vi "ECHOLAB_sweep_BlueMagic_8_LED_robot.vi"() -> ()   [LabVIEW 2014]
uses:
  <vilib>/Analysis/NI_AALBase.lvlib
  <vilib>/Analysis/NI_AALPro.lvlib
  <vilib>/Analysis/2dsp.llb/1D Cross Correlation (DBL).vi
  <vilib>/Analysis/baseanly.llb/Mean (DBL).vi
  <vilib>/DAQmx/write.llb/DAQmx Write (Digital Bool 1Line 1Point).vi
  <vilib>/DAQmx/write.llb/DAQmx Write (Digital 1D Bool NChan 1Samp 1Line).vi
panel:
  out "error out 7":errorcluster
  in  "only one speaker":bool
  in  "Numerisch":i32=6
  in  "Registerkarte":T1(tab)=enum."Statistic"
  in  "?":T2(tab)=enum."Sweep"
  in  "Grundpfad":path=path "C:/Users/Administrator/Documents/New LabView Programms/Aktuelle Programme/Experiment!/Markus/Test_biege_easyIsle"
  in  "Projektname":string="lasttest"
  in  "Lsimp Path":path=path "C:/Users/Administrator/Documents/New LabView Programms/Aktuelle Programme/Experiment!/Markus/Lsimps/Lsimp_EMFI_doubleLayer2"
  out "Projektpfad":path
  in  "EMFI":bool=TRUE
  in  "Sequenz length us":i32=10000
  in  "Sweep Position us":i32=1000
  in  "Fading length us":i32=100
  out "Sweep":waveform(dbl)(graph)={"t0"=timestamp(0 s since 1904-01-01), "dt"=2e-06, "Y"=array[10000 elements]}
  in  "Sweep Dauer us":dbl=3000.0
  in  "Endfrequenz":dbl=30000.0
  in  "Startfrequenz":dbl=160000.0
  in  "Speichern":bool
  out "Active Speaker":bool[](array[boolean])=[FALSE, FALSE, FALSE, FALSE, FALSE, FALSE, FALSE, FALSE, FALSE, FALSE, FALSE, FALSE, TRUE, FALSE]
  out "Current Step":i32=9
  in  "Lautsprecher Winkel 2":dbl[](array[numeric])=[57.5, 62.5, 67.5, 72.5, 77.5, 82.5, 87.5, 92.5, 97.5, 102.5, 107.5, 112.5, 117.5, 122.5]
  in  "?":T3(tab)=enum."Korreliertes Signal 2"
  out "Rohdaten Mic_2":dbl[](graph)
  out "Rohdaten Mic_1":dbl[](graph)
  out "Highpass gefilterte Rohdaten 1":dbl[](graph)
  out "Highpass gefilterte Rohdaten 2":dbl[](graph)
  out "Korreliertes Signal mit richtigem Anfang 1":dbl[](graph)
  out "Mit Sweep korreliert 1":dbl[](graph)
  in  "begin signal 1":dbl=10000.0
  out "Korreliertes Signal mit richtigem Anfang 2":dbl[](graph)
  out "Mit Sweep korreliert 2":dbl[](graph)
  in  "begin signal 2":dbl=10000.0
  out "Verwendete Lsimp":dbl[](graph)=[37.987285423059056, 41.94542933552669, 36.718158358422706, 26.00748307572737, 19.2716180504421, 24.761499073823494, 42.30499601827574, 61.587948563187, 67.89628573083789, 51.70333227535859, 15.399122766613395, -27.68927453387939, -61.37070763335237, -76.15264916698138, -73.86768017091444, -64.72079033459252, -59.52381378965343, -62.88653630335647, -71.76717343532985, -79.45389721021402, -81.22866913949802, -77.36925543013777, -71.79685821069825, -68.16933219563248, -66.83716345038205, -64.88396753245559, -58.77939161586293, -47.22913366886196, -31.960097661366042, -16.007911276056277, -0.957601780562999, 14.83258011472596, 35.88426996664442, 67.42646016772136, 112.61329444376922, 170.32046883201753, 234.13868277323354, 292.7129302295323, 331.46153784141086, 335.73707485805517, 295.22335233505146, 208.6390119317919, 86.97778592958551, -46.80965343474546, -163.0212483502424, -234.6982045240623, -248.3565916317663, -211.17170036320425, -150.16619266006217, -101.95868271871649, -96.40529026626245, -141.58789070049625, -218.28587106890322, -288.03302525625713, -311.67350917905657, -269.0264147906947, -169.00057710982665, -44.606841115389614, 64.01890415431463, 128.6594928873974, 143.66493430186893, 123.6892963416052, 92.1901251937388, 69.13583532468809, 64.83922327141428, 80.91465595446554, 114.10505366272857, 158.17423887163412, 202.9849929659505, 234.17069835907236, 237.13810720723058, 204.90368531355756, 144.26755083610885, 74.11421963653709, 14.839045579973371, -24.61012928577484, -52.16863709716678, -85.0542584663164, -133.37595971808742, -186.99256816490333, -216.89265836020712, -192.62474702620085, -105.2705475364944, 19.88830084818578, 131.07229196653836, 174.9072799253783, 123.9788348833058, -9.122072661395347, -178.45784850808047, -326.4793694986597, -407.4491440952962, -400.941475403144, -312.31821988357115, -165.1330278590582, 7.545121930961784, 169.73077975035375, 288.6320105760493, 342.59757383091426, 329.43731496614197, 269.5355622823815, 198.62746495525653, 151.1277946685444, 142.28248330950265, 160.03536063923315, 172.48295121369566, 147.08158850809662, 70.14025726278376, -44.961580421148035, -164.9711932091802, -253.9338579639399, -289.68706855950416, -271.08402995295086, -214.24499349508537, -142.51142765887988, -76.62533165610529, -29.048182137794647, -2.5152144966053003, 8.879387744009524, 16.999498652431683, 35.028807650487735, 70.9591859098809, 121.51231551074474, 170.52550094534286, 194.6168672600115, 174.70853553953242, 107.51186045471589, 9.93561022984685, -87.01517468482572, -152.02697733843473, -167.43181691881233, -135.84534566440934, -76.63424130617673, -15.304023561933974, 27.73181681265263, 43.48100822634696, 34.20774270023911, 9.028054419071426, -21.094648548475305, -46.562847934060166, -60.39229615626998, -58.61648097387942, -40.720888785491965, -9.95678133454292, 27.198727840329127, 62.78429492138909, 89.75636837754168, 103.97627526024421, 104.94515156439942, 95.17354586658846, 78.67523010824826, 59.256086140600914, 39.14916197776178, 18.419707567058776, -4.53429131695286, -31.359167324869112, -61.60716713863444, -91.31357632662373, -113.5222858413143, -121.02690136101434, -110.10016494050913, -83.00220288733615, -47.49118008118892, -13.322545050646244, 12.316883061252692, 27.737392500670154, 36.38229758518521, 43.65244700708752, 53.12187538151082, 64.48349513224547, 74.14700753033969, 77.60736295621001, 71.80331292821236, 56.17513240504583, 32.37375911823534, 3.4627367567873555, -26.62897321273065, -53.397178059119526, -72.34957116923633, -80.22839594278574, -76.41884765260448, -63.53246629100458, -46.440467539101725, -30.051069869735283, -17.082827718919397, -7.188938774909889, 2.0994401876032778, 13.343105063752096, 27.432584546910252, 43.08171772566773, 57.587134526822325, 68.0662292444963, 72.33213728362517, 69.13204626316582, 58.08493838266445, 39.7682572566104, 16.002080433379952, -10.069811728438523, -34.5306095944581, -53.8364889717854, -65.97272873380305, -70.90309347902996, -70.02677876043627, -65.03196685626713, -56.90758277963846, -45.69501643915526, -31.00235289689016, -12.805913828058124, 8.013068875792442, 29.644160069832875, 49.706586339083785, 65.72366452061605, 75.56557454467972, 77.8751474823423, 72.48313804653267, 60.64901799215318, 44.85647944539737, 28.053216272045916, 12.592101934969236, -0.5703833046869773, -11.92788800291775, -22.68227095779246, -33.678613480551, -44.69092768297345, -54.460430330636825, -61.351280097982695, -64.10659971309258, -62.226391914044754, -55.86269279903715, -45.52248460302857, -31.930615670932838, -16.144321341606098, 0.3192571896456796, 15.651291021180189, 28.259121968674897, 37.307148605525796, 42.86896311084485, 45.52674876328166, 45.68907117249621, 43.1533923702947, 37.285299525259305, 27.717818644463748, 15.063835342580322, 1.09861362859763, -11.761034684139855, -21.362230547589427, -26.545860965660452, -27.311966112040114, -24.449178789685256, -18.98880063520781, -11.859596605121695, -3.8566927215703863, 4.246542650360977, 11.681910293034626, 17.83766248205442, 22.428960778401663, 25.480209919729468, 27.078861865530516, 27.08775142595211, 25.082005453718555, 20.611753000725564, 13.626659246561587, 4.7425311670550885, -4.869942969188056, -13.919586156575697, -21.471781523790362, -27.177548910451407, -31.16182125158828, -33.71583021036854, -35.03910551569061, -35.16954647736422, -34.06207997379421, -31.669590588025734, -27.936554105228137, -22.75141917097973, -15.980520596397886, -7.639329094944579, 1.8899819246897778, 11.769595911840018, 20.859044110038674, 28.056029628887828, 32.627847523818204, 34.35154124141151, 33.42281412422663, 30.256602385756544, 25.346837423716195, 19.256450690601064, 12.661021482984339, 6.318294154753728, 0.912547672939884, -3.13874461051835, -5.76817117503621, -7.15697915173641, -7.522403709934467, -6.960713149988033, -5.465938798812448, -3.0917352098321413, -0.09624096730401532, 3.0748575670448757, 5.970285329410185, 8.33003766291407, 10.126408347639087, 11.40559072656139, 12.06406962932657, 11.756856138530953, 10.033353177332586, 6.611505107116842, 1.5840530992770214, -4.594870237638631, -11.322520610248993, -18.082087377026, -24.521473842257514, -30.34447353803086, -35.150092644557205, -38.400157160262964, -39.57989702216926, -38.43148546041212, -35.06667472234177, -29.850930108971063, -23.142794630831233, -15.106002216192778, -5.765961157179861, 4.719486173324453, 15.78972267144523, 26.45011877168526, 35.54746915313663, 42.18800189416256, 46.024055317696046, 47.23280922339901, 46.23648737352134, 43.39003268668904, 38.85941230891154, 32.74295226898982, 25.29262513752641, 17.025656379837578, 8.623949422155569, 0.7042607056616654, -6.355400409638805, -12.406264834922581, -17.370160143207055, -21.092711794336847, -23.35391752325315, -24.03506410806453, -23.295367971810453, -21.592699300181494, -19.50292468346278, -17.45795729745628, -15.591256485359558, -13.80111204093922, -11.971363960105585, -10.17454538585567]
  out "error out 2":errorcluster
  in  "Datenbank? R1-M1":bool=TRUE
  in  "Datenbank? R1-M2":bool=TRUE
  in  "Datenbank? R2-M1":bool=TRUE
  in  "Datenbank? R2-M2":bool=TRUE
  in  "Datenbank? R3-M1":bool=TRUE
  in  "Datenbank? R3-M2":bool=TRUE
  in  "Pfad? R1-M1":path=path "C:/Users/Administrator/Documents/New LabView Programms/Aktuelle Programme/Experiment!/HuanSubVIs/S70-21_M1.csv"
  in  "Pfad? R1-M2":path=path "C:/Users/Administrator/Documents/New LabView Programms/Aktuelle Programme/Experiment!/HuanSubVIs/S70-21_M2.csv"
  in  "Pfad? R2-M1":path=path "C:/Users/Administrator/Documents/New LabView Programms/Aktuelle Programme/Experiment!/HuanSubVIs/S50-20_M1.csv"
  in  "Pfad? R2-M2":path=path "C:/Users/Administrator/Documents/New LabView Programms/Aktuelle Programme/Experiment!/HuanSubVIs/S50-20_M2.csv"
  in  "Pfad? R3-M1":path=path "C:/Users/Administrator/Documents/New LabView Programms/Aktuelle Programme/Experiment!/HuanSubVIs/S35-10_M1.csv"
  in  "Pfad? R3-M2":path=path "C:/Users/Administrator/Documents/New LabView Programms/Aktuelle Programme/Experiment!/HuanSubVIs/S35-10_M2.csv"
  in  "Gap Refl2 (samples)":dbl=62.0
  in  "Gap Refl1 (samples)":dbl=85.0
  in  "Gap Refl3 (samples)":dbl=41.0
  in  "MaxtPeak miltiplication \nfactor -R1":dbl=15.0
  in  "MaxtPeak miltiplication\n factor R3":dbl=25.0
  in  "MaxtPeak miltiplication\n factor -R2":dbl=50.0
  in  "Grenz Ampulitude-R3":dbl=80.0
  in  "Grenz Ampulitude-R1":dbl=100.0
  in  "Grenz Ampulitude-R2":dbl=100.0
  out "Refl_1":dbl[][](graph)
  out "Refl_3":dbl[][](graph)
  in  "Stopabstand 1":dbl=30.0
  out "Max. Wert Refl_1":dbl=0.00024072035967195873
  in  "Stopabstand 2":dbl=30.0
  out "Abstand-Array-Refl 2":dbl=38.09710163220162
  in  "turn left/right?":bool=TRUE
  out "Max. Wert Refl_2":dbl=0.0023395203738088097
  in  "Stopabstand 3":dbl=30.0
  out "Abstand-Array-Refl 3":dbl=62.91468799787438
  in  "LED turn on?":bool=TRUE
  out "Max. Wert Refl_3":dbl=0.0018103910057642178
  out "probability":dbl[][](graph)=[[3.0000000000000004e-05, 5.000000000000001e-05, 7.000000000000001e-05, 9e-05, 0.00011, 0.0001300124738367786, 0.00023072035967195873, 0.00025072035967195873], [3.0000000000000004e-05, 5.000000000000001e-05, 7.000000000000001e-05, 9e-05, 0.0017493906595402342, 0.0017803910057642178, 0.0018003910057642178, 0.0018203910057642179], [0.00038194151602209035, 0.0009686688450150448, 0.0022439203760585267, 0.004143838935916074, 0.005245931301535438, 0.005272342187251083, 0.002320526795117191, 0.0023585139525004284]]
  out "probability/distance":dbl[][](graph)=[[1.8750000000000003e-06, 5.891036022775227e-06, 6.000006000006e-11, 8.000008000008e-11, 1.0000010000010001e-10, 3.239128915113618e-06, 4.868667316483549e-06, 8.424336383279796e-06], [1.8750000000000003e-06, 5.891036022775227e-06, 6.000006000006e-11, 8.000008000008e-11, 1.185535180537081e-05, 2.5560005321415227e-05, 2.593027246994507e-05, 2.9887064473399943e-05], [5.616787000324858e-06, 1.1108824384371127e-05, 3.0643367217874765e-05, 7.270750187692021e-05, 0.0001283583707298027, 0.00018749870693041687, 9.480098082220174e-05, 6.766626049238367e-05]]
  in  "robotControl":bool
  out "Actions?":bool=TRUE
  in  "x links Refl1":i32=200
  in  "y links Refl1":i32=500
  out "x/y":dbl=1e-05
  out "gefahrene (cm)":dbl=59.86920617947912
  out "time diff (s)":dbl=3.314115524291992
  out "gefahren(mm)":dbl=84.43606431317178
  in  "Velocity":dbl=4000.0 format="%#_13g"
  in  "origin Y(cm)":dbl=-10.0 format="%#_13g"
  in  "Velocity (mm per sec)":dbl=40.0 format="%#_13g"
  in  "robot aktiv":bool
  in  "Lineareinheit aktiv":bool=TRUE
  in  "x-move (mm)":dbl=8000.0
  out "R1-Action":bool
  out "R2-Action":bool
  out "R3-Action":bool
  out "Abstand-Array-Refl1":dbl=28.64430745806648
  in  "Sigma-R3":dbl=1.8
  in  "Sigma-R2":dbl=1.5
  in  "Sigma-R1":dbl=1.0
  out "Abstand-Array-Refl3\n(in y Richtung)":dbl=60.57440025183806
  out "Abstand-Array-Refl2\n(in y Richtung)":dbl=34.57440025183806
  out "Abstand-Array-Refl1\n(in y Richtung)":dbl=28.574400251838057
  out "y_R3":i32=112
  out "x_R3":i32=83
  out "y_R1":i32=80
  out "x_R1":i32=102
  out "y_R2":i32=86
  out "x_R2":i32=82
  out "Refl_2":dbl[][](graph)
  out "Signalverlaufsgraph 3":dbl[][](graph)
  out "korriliertes Singnal":dbl[](graph)
  in  "Mic. 1      /      Mic. 2":bool
  in  "LS auswählen":i32=11
  in  "Standard Gap eingeben":dbl=85.0
  out "Locations":dbl[](array[numeric])
  out "distanceMatrix":dbl[][](array[numeric])
  out "Array 2":dbl[](array[numeric])
  out "HS":bool
  in  "MaxtPeak miltiplication factor":dbl=50.0
  in  "Stopp 2":bool
  in  "Message":string="60;0;15"
  out "error out 6":errorcluster
  out "error out 5":errorcluster
  # "Nein"
  # "Ja"
  # "1     2     3     4     5     6     7     8     9    10   11   12   13   14"
  # "Polaroid"
  # "orange 70 mm"
  # "blau 50 mm"
  # "gruen 35 mm"
  # "green"
  # "orange"
  # "blau"
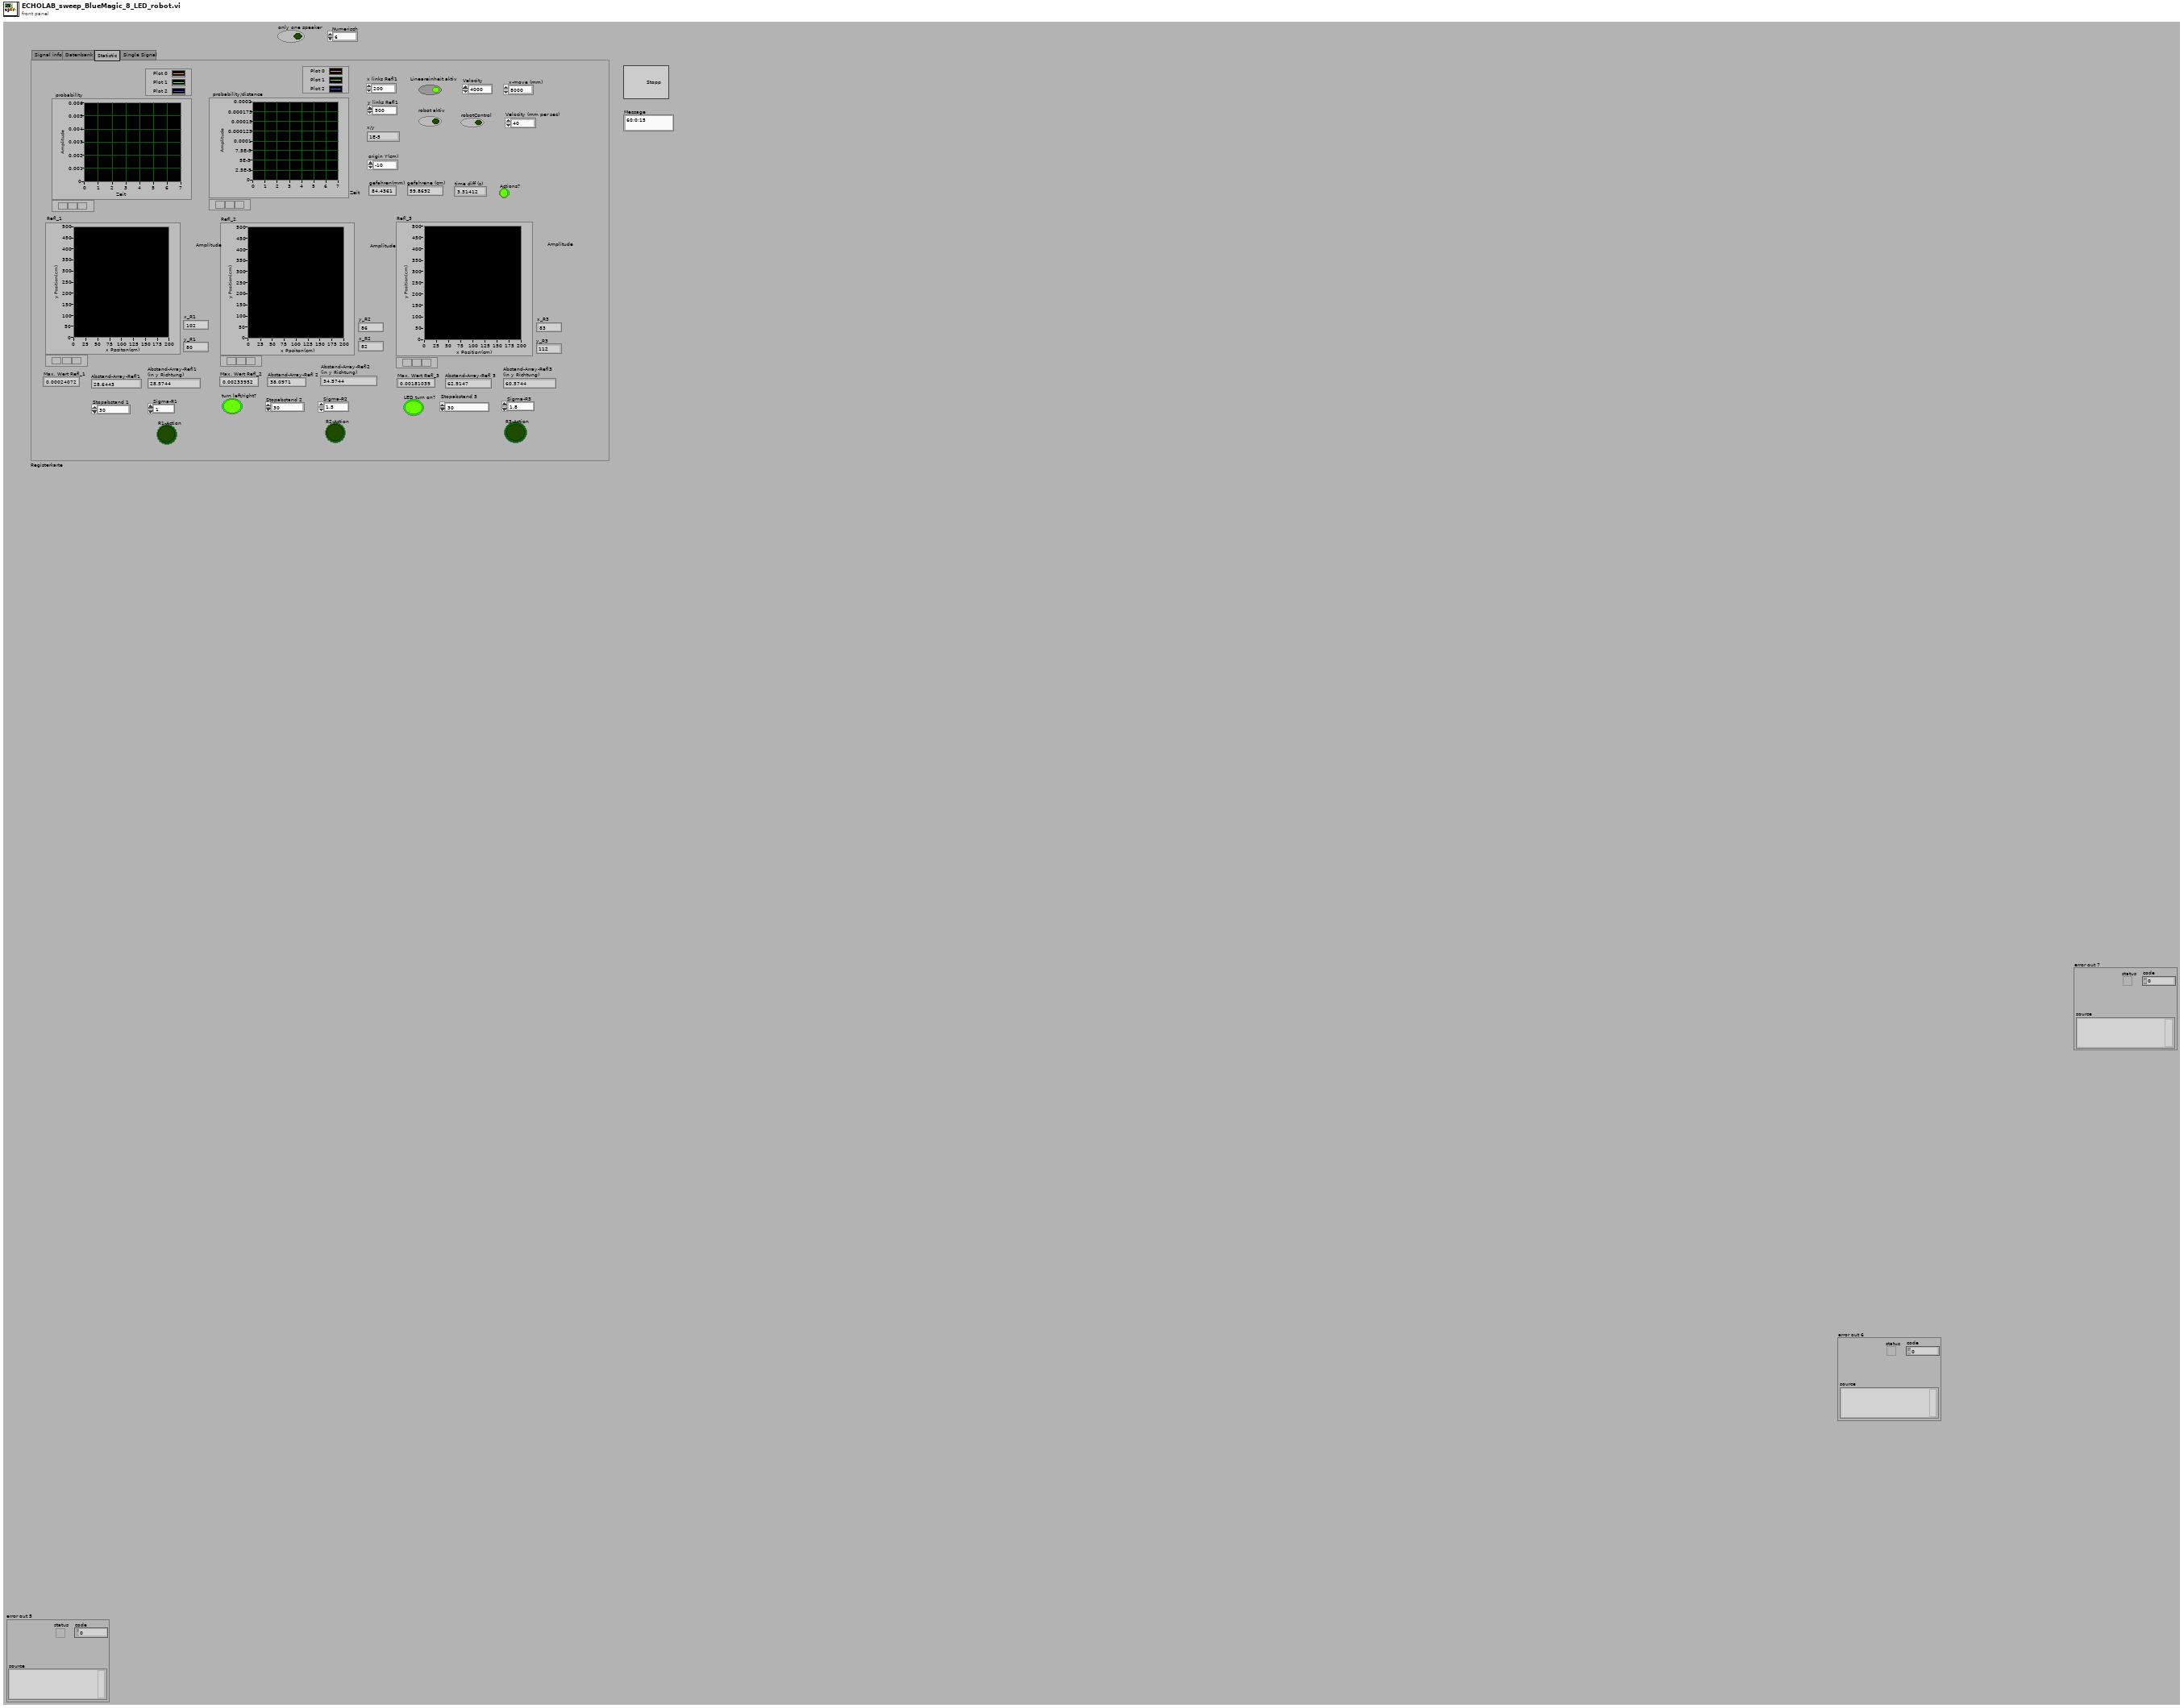
[diagram p1: front panel]
types:
  T1 = enum32{"Signal info", "Datenbank", "Statistic", "Single Signal"}
  T2 = enum32{"Daten einlesen und speichern", "Sweep", "HK", "Winkel & Korrektur"}
  T3 = enum32{"Rohdaten", "Rohdaten HP", "Korreliertes Signal 1", "Korreliertes Signal 2", "Intensity Graphs", "Lsimp", "Errors"}
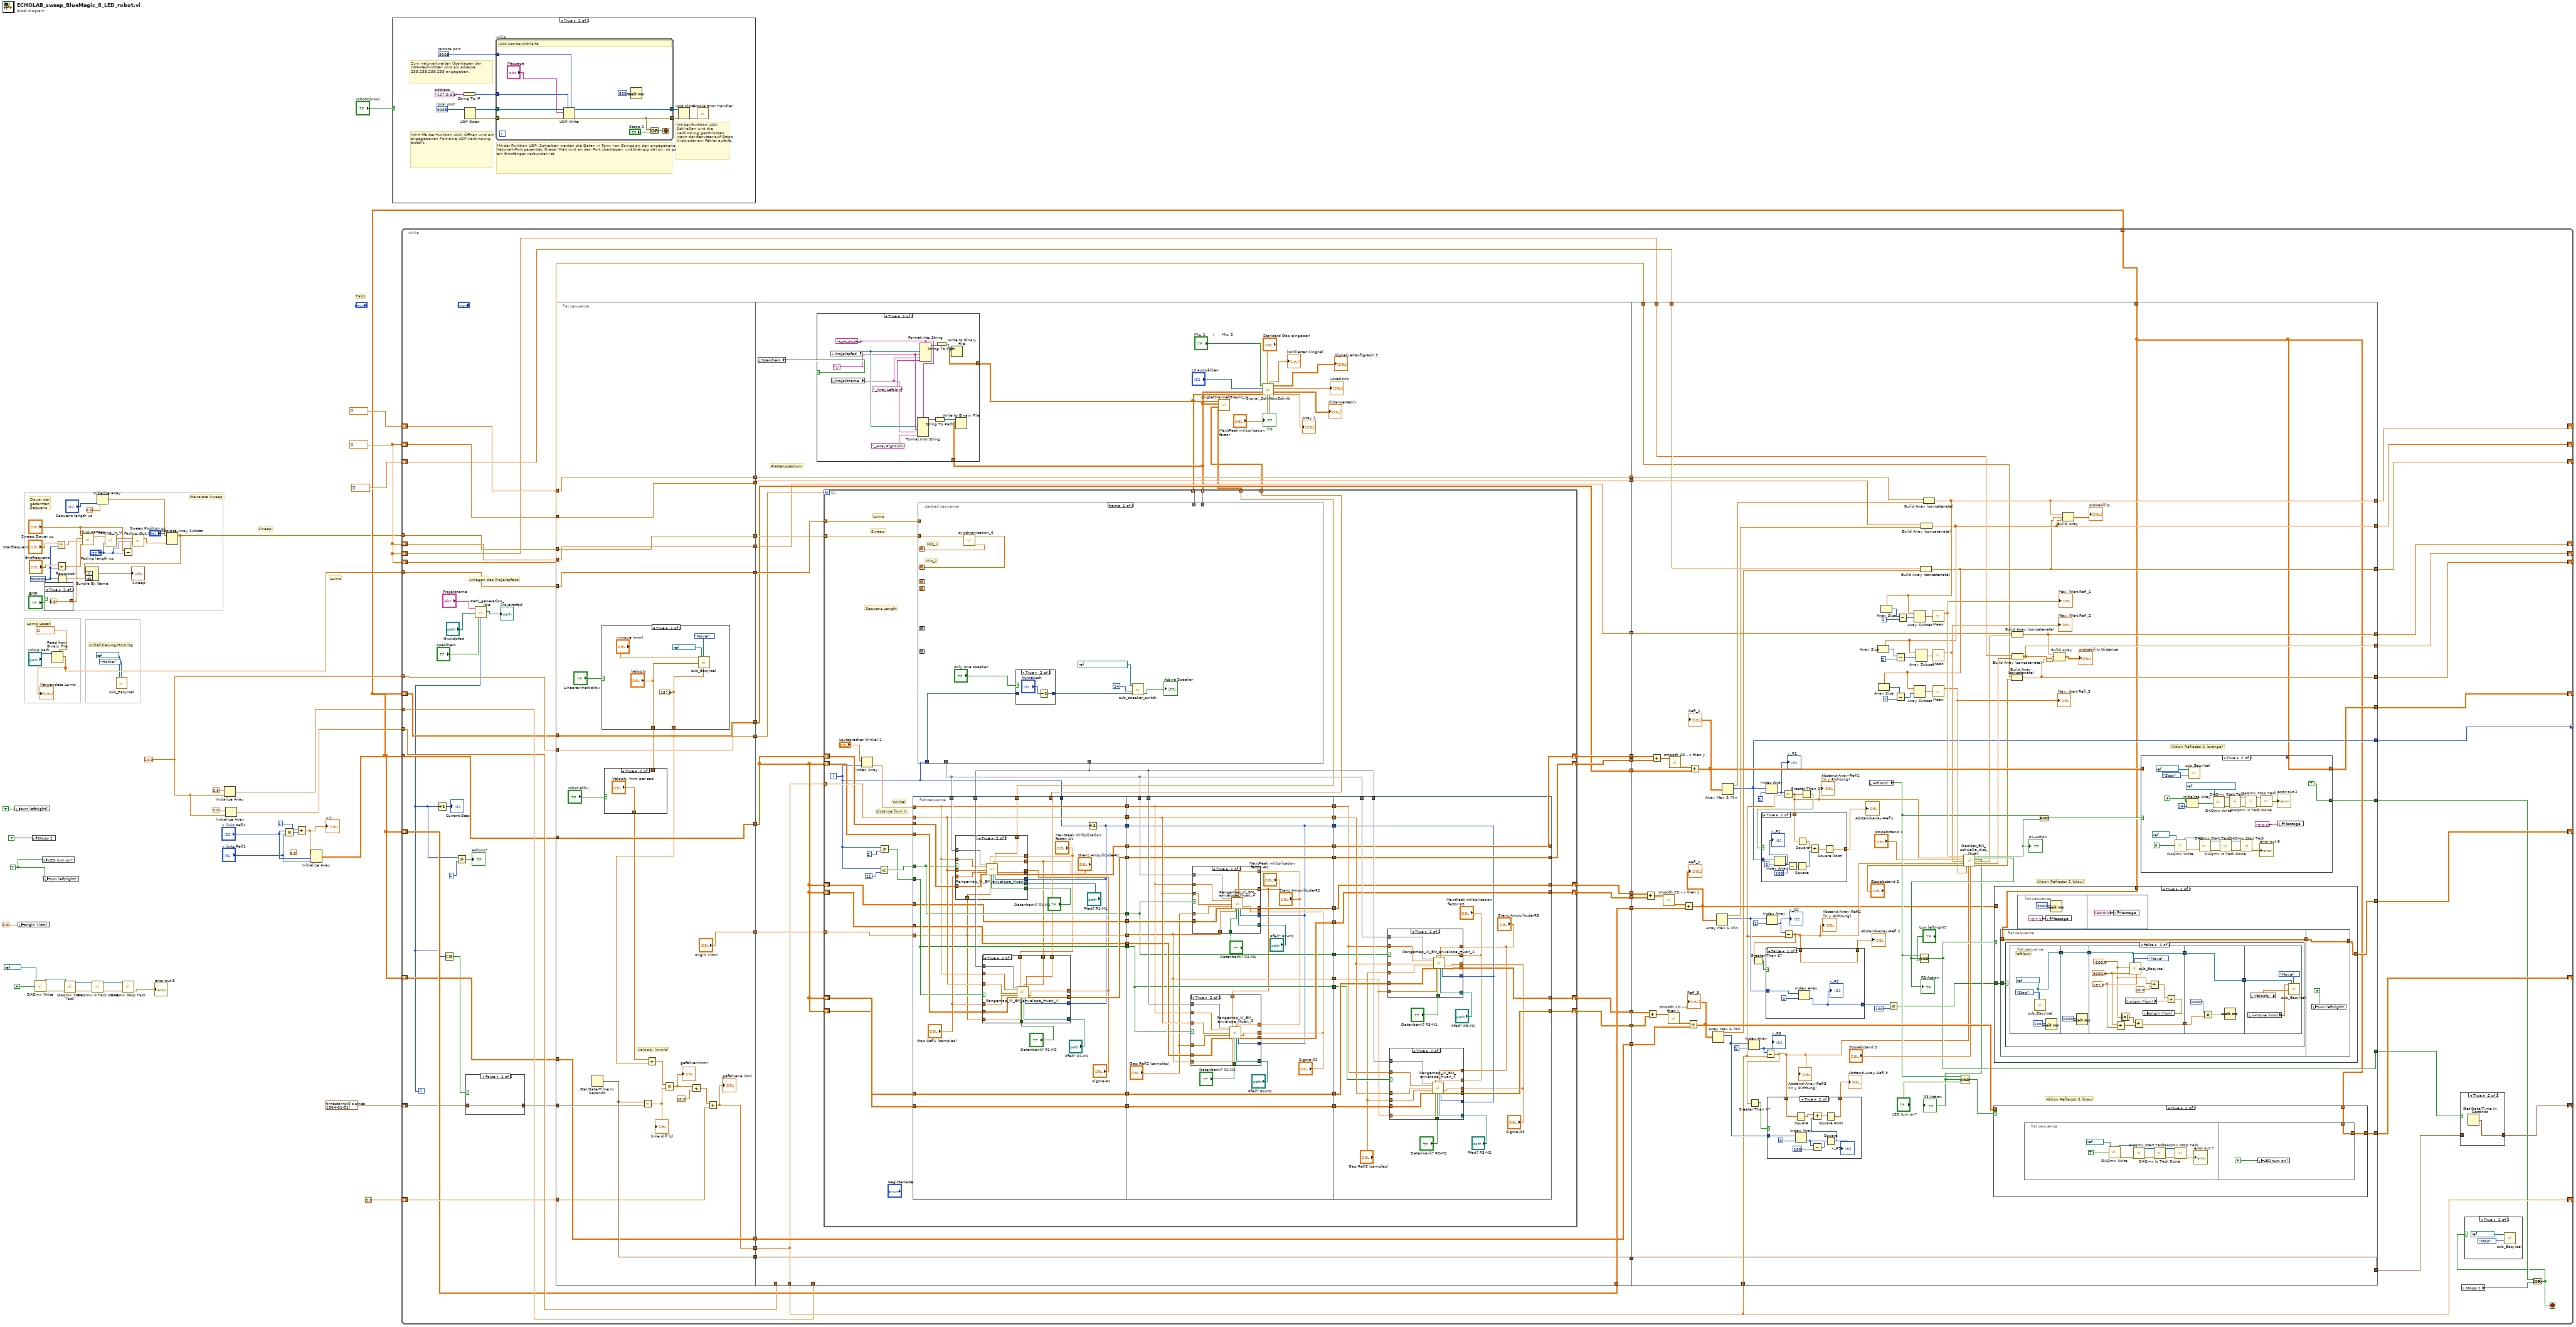
[diagram p0: block diagram]
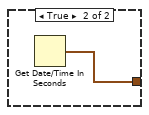
[diagram p5: hidden frame]
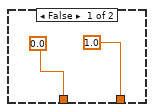
[diagram p7: hidden frame]
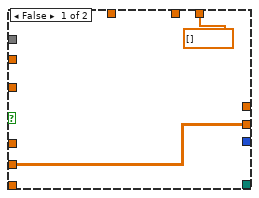
[diagram p9: hidden frame]
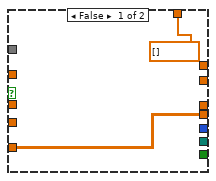
[diagram p10: hidden frame]
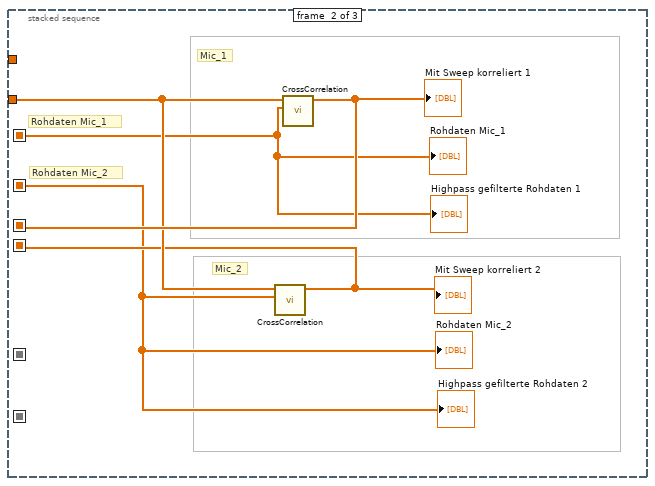
[diagram p16: hidden frame]
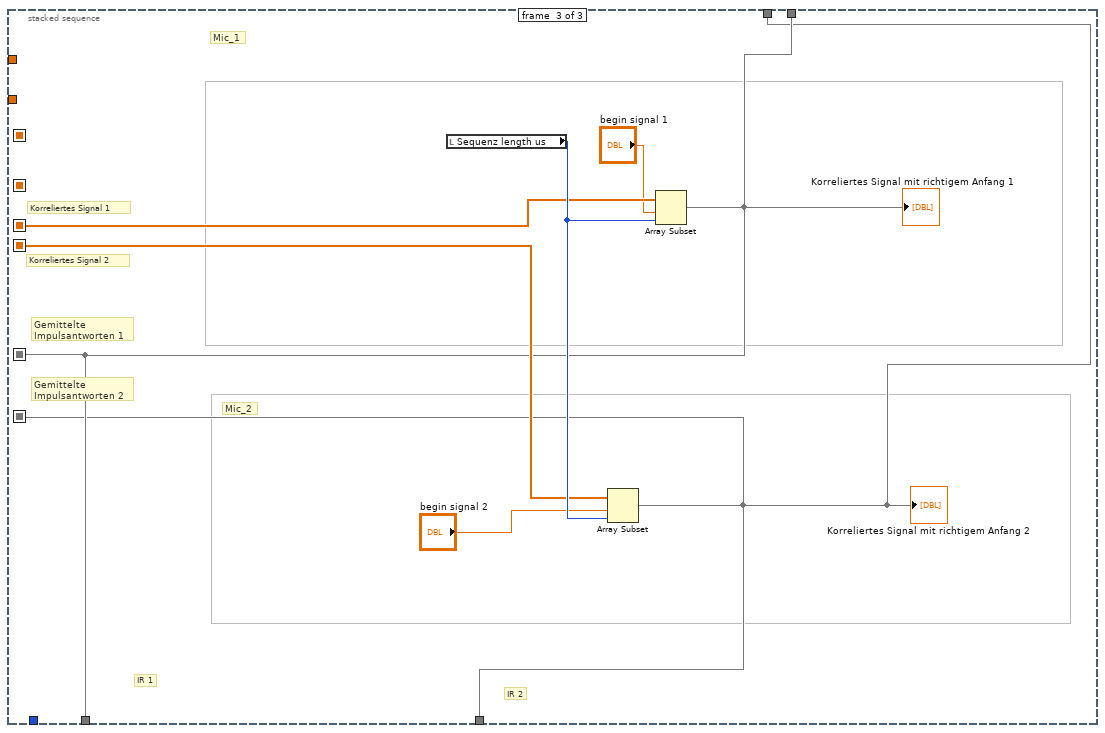
[diagram p17: hidden frame]
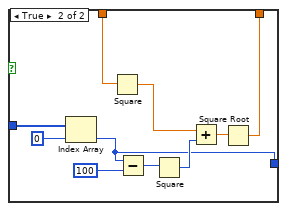
[diagram p19: hidden frame]
diagram:
  w15 = dbl[] []
  w21 = TRUE
  (unwired) 0.0 ("Element")
  w30 = 14.0 ("Anzahl Lautsprecher")
  w48 = 500000
  # "Sweep"
  # "Lsimp"
  # "Initialisierung/Homing"
  # "Dauer der\ngesamten\nSequenz"
  # "Generate Sweep"
  # "Tabs"
  # "Lsimp Lesen"
  n1 = local write "turn left/right?"(TRUE ("x < y?")) -> ()
  n2 = local write "origin Y(cm)"(0.0 ("origin(cm) Y")) -> ()
  n3 = local write "Stopp 2"(FALSE) -> ()
  n4 = call-poly <vilib>:"DAQmx Write.vi"("task/channels in"=refnum<k21> "LED", "data"=FALSE) -> ("task out"=w14:refnum<k21>, "error out"=w13:errorcluster)  [unwired: 11 in, 1 out]
  n5 = local write "LED turn on?"(w21) -> ()
  n6 = local write "turn left/right?"(w21) -> ()
  n7 = case shown="True" "EMFI" {
    tunnel: [1 9.0 ("amplitude")] -> w34
    frame False {
    }
    frame True {
    }
  }
  n8 = Read from Binary File(5:dbl[] [], 11:"Lsimp Path") -> (2:w53:dbl[])  [unwired: 4 in, 3 out]
  "Verwendete Lsimp" <- w53
  n9 = Divide(x="Startfrequenz", y=w48) -> (x/y=w51:dbl)
  n10 = Divide(x="Endfrequenz", y=w48) -> (x/y=w49:dbl)
  n11 = Reciprocal(x=w48) -> (1/x=w47:dbl)
  n12 = call <vilib>:"DAQmx Start Task.vi"("task/channels in"=w14, "error in"=w13) -> ("task out"=w12:refnum<k21>, "error out"=w11:errorcluster)  [unwired: 12 in]
  n13 = call <vilib>:"Chirp Pattern.vi"("f2"=w49, "f1"=w51, "amplitude"=w34, "samples"="Sweep Dauer us") -> ("Chirp Pattern"=w44:dbl[])  [unwired: 1 out]
  n14 = call <vilib>:"DAQmx Is Task Done.vi"("task/channels in"=w12, "error in"=w11) -> ("task out"=w10:refnum<k21>, "error out"=w9:errorcluster)  [unwired: 11 in, 1 out]
  n15 = Initialize Array(0.0 ("element"), "Sequenz length us") -> (w43:dbl[])
  n16 = call "Fading_In_VI.vi"("Input Array"=w44, "Fading Index"="Fading length us") -> ("Rising Array"=w42:dbl[])  [unwired: 12 in, 1 out]
  n17 = call "sub_EasyIsel.vi"("VISA resource name"=refnum<visa-resource-name> "COM4", "Mode"=enum16{"Position", "Move", "Stop", "Home"}."Home") -> ()  [unwired: 14 in, 4 out]
  n18 = Subtract(x="Sweep Dauer us", y="Fading length us") -> (x-y=w40:dbl)
  n19 = call <vilib>:"DAQmx Stop Task.vi"("task/channels in"=w10, "error in"=w9) -> ("error out"=→"error out 5":errorcluster)  [unwired: 12 in, 1 out]
  n20 = call "Fading_Out_VI.vi"("Input Array"=w42, "Fading length"="Fading length us", "Fading Index"=w40) -> ("Faded Array"=w41:dbl[])  [unwired: 11 in, 1 out]
  n21 = Replace Array Subset(array=w43, new element=w41, index="Sweep Position us") -> (w4:dbl[])
  n22 = Bundle By Name("Y"=w4, "dt"=w47) -> (→"Sweep":waveform(dbl))  [unwired: 1 in]
  n23 = Initialize Array(0.0, w30) -> (w32:dbl[])
  n24 = Initialize Array(0.0, w30) -> (w29:dbl[])
  n25 = Multiply(x="x links Refl1", y="y links Refl1") -> (x*y=w27:i32)
  n26 = Divide(x=1, y=w27) -> (x/y=w23:dbl)
  "x/y" <- w23
  n27 = Initialize Array(w23, "x links Refl1", "y links Refl1") -> (w17:dbl[][])
  n28 = case shown="True" "robotControl" {
    frame False {
    }
    frame True {
      w58 = u16 5005  # remote port
      w59 = u16 5005  # local port
      w64 = "127.0.0.1"  # address
      # "Zum netzwerkweiten Übertragen der UDP-Nachrichten wird als Adresse 255.255.255.255 angegeben."
      # "Mit der Funktion UDP: Schließen wird die Verbindung geschlossen, wenn der Benutzer auf Stopp klickt oder ein Fehler auftritt."
      # "Mit der Funktion UDP: Schreiben werden die Daten in Form von Strings an den angegebenen Netzwerk-Port gesendet. Dieser Wert wird an den Port übertragen, unabhängig davon, ob gerade ein Empfänger verbunden ist."
      # "Mit Hilfe der Funktion UDP: Öffnen wird am angegebenen Port eine UDP-Verbindung erstellt."
      n29 = String To IP(1:w64) -> (0:w62:u32)
      n30 = UDP Open(11:w59) -> (port=w61:refnum<k16>, 0:w60:errorcluster)  [unwired: 4 in, 1 out]
      n31 = while {
        tunnel: [w71] -> w65
        tunnel: w61 -> [w76]
        tunnel: w60 -> [w75]
        tunnel: [w72] -> w66
        tunnel: w62 -> [w70]
        tunnel: w58 -> [w68]
        stop <- w74 stop-if-true
        # "UDP-Sender-Schleife"
        n32 = UDP Write(address=w70, port or service name=w68, connection ID=w76, data in="Message", 8:w75) -> (error out=w71:errorcluster, 3:w72:refnum<k16>)  [unwired: 1 in]
        n33 = Wait (ms)(milliseconds to wait=u32 500) -> ()  [unwired: 1 out]
        n34 = Or(x=w71, y="Stopp 2") -> (x .or. y?=w74:bool)
      }
      n35 = UDP Close(connection ID=w66, 8:w65) -> (error out=w63:errorcluster)  [unwired: 1 out]
      n36 = call <vilib>:"Simple Error Handler.vi"("error in (no error)"=w63) -> ()  [unwired: 4 in, 5 out]
    }
  }
  n37 = while {
    tunnel: w30 -> [w141]
    tunnel: w53 -> [w146]
    tunnel: w4 -> [w87]
    tunnel: w32 -> [w142]
    tunnel: w29 -> [w140]
    shift-right: [w97] -> _
    shift-left: timestamp(0 s since 1904-01-01) ("seconds since 1Jan1904") -> [w102]
    shift-right: [w81] -> _
    shift-left: 0.0 -> [w134]
    tunnel: [w83] -> _ mode=indexing
    shift-right: [w86] -> _
    shift-left: w17 -> [w117]
    shift-right: [w126] -> _
    shift-left: dbl[] [] -> [w127]
    shift-right: [w128] -> _
    shift-left: w15 -> [w125]
    tunnel: w17 -> [w119]
    shift-right: [w116] -> _
    shift-left: w17 -> [w114]
    shift-right: [w85] -> _
    shift-left: w17 -> [w110]
    shift-right: [w105] -> _
    shift-left: dbl[] [] -> [w104]
    tunnel: w17 -> [w100]
    shift-right: [w82] -> _
    shift-left: w15 -> [w94]
    shift-right: [w96] -> _
    shift-left: w15 -> [w91]
    shift-right: [w95] -> _
    shift-left: w15 -> [w90]
    i -> [w88]
    stop <- w78 stop-if-true
    # "Anlegen des Projektpfads"
    n38 = Increment(x=w88) -> (x+1=→"Current Step":i32)
    n39 = Equal To 0?(x=w88) -> (x = 0?=w103:bool)
    n40 = Greater?(x=w88, y=1) -> (0:→"Actions?":bool)
    n41 = case shown="False" w103 {
      tunnel: w102 -> [w151 _]
      tunnel: [w151 w152] -> w101
      frame False {
      }
      frame True {
        n42 = Get Date/Time In Seconds() -> (seconds since 1Jan1904=w152:timestamp)
      }
    }
    n43 = call "Path_generation_isle.vi"("Projektname"="Projektname", "Basis-Pfad"="Grundpfad", "Pfad erstellen ? [T]"="Speichern", "Revison"=w88) -> ("Erstellter Pfad"=→"Projektpfad":path)  [unwired: 11 in, 4 out]
    n44 = flat-sequence {
      tunnel: w87 -> [w174]
      tunnel: w146 -> [w175]
      tunnel: w141 -> [w176]
      tunnel: [w176] -> w145
      tunnel: [w175] -> w144
      tunnel: [w174] -> w143
      tunnel: [w170] -> w137
      tunnel: w101 -> [w169]
      tunnel: [w153] -> w135
      tunnel: w134 -> [w155]
      tunnel: w127 -> [w167]
      tunnel: w125 -> [w166]
      tunnel: [w167] -> w124
      tunnel: [w166] -> w122
      tunnel: [w165] -> w120
      tunnel: w119 -> [w165]
      tunnel: [w164] -> w115
      tunnel: w114 -> [w164]
      tunnel: w110 -> [w163]
      tunnel: [w163] -> w109
      tunnel: ["origin Y(cm)"] -> w99
      tunnel: w94 -> [w161]
      tunnel: [w161] -> w93
      tunnel: w145 -> [w215]
      tunnel: w144 -> [w219]
      tunnel: w143 -> [w214]
      tunnel: w142 -> [_]
      tunnel: w140 -> [_]
      tunnel: [w217] -> w139
      tunnel: [w216] -> w138
      tunnel: w137 -> [w190]
      tunnel: [w190] -> w136
      tunnel: w135 -> [w191]
      tunnel: [w213] -> w130
      tunnel: [w200] -> w129
      tunnel: w124 -> [w212]
      tunnel: [w212] -> w123
      tunnel: w122 -> [w211]
      tunnel: [w211] -> w121
      tunnel: w120 -> [w205]
      tunnel: [w210] -> w118
      tunnel: w117 -> [w210]
      tunnel: w115 -> [w209]
      tunnel: [w209] -> w113
      tunnel: [w208] -> w112
      tunnel: [w207] -> w111
      tunnel: w109 -> [w206]
      tunnel: [w206] -> w108
      tunnel: w99 -> [w204]
      tunnel: w93 -> [w203]
      tunnel: [w203] -> w92
      tunnel: [w191] -> w81
      tunnel: w139 -> [w503]
      tunnel: w138 -> [w557]
      tunnel: w136 -> [w523]
      tunnel: [w523] -> w98
      tunnel: w81 -> [w486]
      tunnel: w130 -> [w560]
      tunnel: w129 -> [w502]
      tunnel: [w529] -> w126
      tunnel: [w474] -> w128
      tunnel: w123 -> [w562]
      tunnel: w121 -> [w561]
      tunnel: [w526] -> w86
      tunnel: w118 -> [w501]
      tunnel: [w527] -> w116
      tunnel: w113 -> [w554]
      tunnel: w112 -> [w550]
      tunnel: w111 -> [w549]
      tunnel: [w524] -> w85
      tunnel: w108 -> [w546]
      tunnel: [w473] -> w105
      tunnel: w104 -> [w545]
      tunnel: w100 -> [w472]
      tunnel: [w508] -> w82
      tunnel: [w476] -> w96
      tunnel: [w475] -> w95
      tunnel: w92 -> [w507]
      tunnel: w91 -> [w477]
      tunnel: w90 -> [w506]
      tunnel: [w505] -> w84
      tunnel: [w485] -> w83
      tunnel: [w498] -> w79
      frame #0 {
        # "Velocity (mm/s)"
        n45 = Get Date/Time In Seconds() -> (seconds since 1Jan1904=w170:timestamp)
        n46 = case shown="True" "Lineareinheit aktiv" {
          tunnel: [0.0 "Velocity"] -> w158
          tunnel: [1.0 w182] -> w156
          frame False {
          }
          frame True {
            w182 = 157.0 ("Steps/mm (x)")
            n47 = call "sub_EasyIsel.vi"("x-Position"="x-move (mm)", "Velocity (x)"="Velocity", "VISA resource name"=refnum<visa-resource-name> "COM4", "Mode"=enum16{"Position", "Move", "Stop", "Home"}."Move", "Steps/mm (y)"=w182) -> ()  [unwired: 11 in, 4 out]
          }
        }
        n48 = case shown="True" "robot aktiv" {
          tunnel: w158 -> [w177 _]
          tunnel: [w177 "Velocity (mm per sec)"] -> w157
          frame False {
          }
          frame True {
          }
        }
        n49 = Subtract(x=w170, y=w169) -> (x-y=w173:dbl)
        "time diff (s)" <- w173
        n50 = Divide(x=w157, y=w156) -> (x/y=w154:dbl)
        n51 = Multiply(x=w154, y=w173) -> (x*y=w172:dbl)
        "gefahren(mm)" <- w172
        n52 = Divide(x=w172, y=10.0) -> (x/y=w168:dbl)
        n53 = Add(x=w168, y=w155) -> (x+y=w153:dbl)
        "gefahrene (cm)" <- w153
      }
      frame #1 {
        # "Plattenspektrum"
        n54 = local read "Speichern"() -> (w218:bool)
        n55 = for {
          N: w215 -> [_]
          tunnel: w219 -> [w284]
          tunnel: w214 -> [w238]
          tunnel: [w283] -> w199 mode=indexing
          tunnel: [w282] -> w198 mode=indexing
          shift-right: [w237] -> w217
          shift-left: w205 -> [w279]
          shift-right: [w252] -> w216
          shift-left: w205 -> [w278]
          tunnel: w191 -> [w280]
          shift-right: [w251] -> w213
          shift-left: w205 -> [w277]
          shift-right: [w250] -> w200
          shift-left: w205 -> [w276]
          shift-right: [w249] -> w208
          shift-left: w205 -> [w275]
          shift-right: [w248] -> w207
          shift-left: w205 -> [w274]
          tunnel: w204 -> [w242]
          tunnel: [w240] -> w202 mode=indexing
          tunnel: [w239] -> w201 mode=indexing
          i -> [w235]
          # "distance from X"
          # "Winkel"
          # "Lsimp"
          # "Sweep"
          # "Sequenz Length"
          n56 = Index Array(array="Lautsprecher Winkel 2", index=w235) -> (element=w281:dbl)
          n57 = Less?(x=w235, y=11) -> (x < y?=w245:bool)
          n58 = Greater?(x=w235, y=2) -> (0:w244:bool)
          n59 = flat-sequence {
            tunnel: w281 -> [w294]
            tunnel: w280 -> [w306]
            tunnel: w279 -> [w310]
            tunnel: w278 -> [w309]
            tunnel: w277 -> [w301]
            tunnel: w276 -> [w300]
            tunnel: w275 -> [w299]
            tunnel: w274 -> [w298]
            tunnel: w236 -> [w307]
            tunnel: w243 -> [w308]
            tunnel: w245 -> [w303]
            tunnel: w244 -> [w302]
            tunnel: [w294] -> w271
            tunnel: [w306] -> w270
            tunnel: [w305] -> w268
            tunnel: [w304] -> w267
            tunnel: [w303] -> w265
            tunnel: [w302] -> w264
            tunnel: [w301] -> w262
            tunnel: [w300] -> w261
            tunnel: [w299] -> w256
            tunnel: [w298] -> w254
            tunnel: w242 -> [w297]
            tunnel: [w297] -> w241
            tunnel: [w296] -> w240
            tunnel: [w295] -> w239
            tunnel: w235 -> [w291]
            tunnel: [w288] -> w234
            tunnel: w271 -> [w354]
            tunnel: w270 -> [w367]
            tunnel: w268 -> [w363]
            tunnel: w267 -> [w362]
            tunnel: [w354] -> w266
            tunnel: w265 -> [w358]
            tunnel: w264 -> [w357]
            tunnel: [w367] -> w263
            tunnel: w262 -> [w366]
            tunnel: w261 -> [w365]
            tunnel: w243 -> [w353]
            tunnel: w236 -> [w364]
            tunnel: [w363] -> w260
            tunnel: [w362] -> w259
            tunnel: [w361] -> w258
            tunnel: [w360] -> w257
            tunnel: w256 -> [w356]
            tunnel: [w356] -> w255
            tunnel: w254 -> [w359]
            tunnel: [w359] -> w253
            tunnel: [w358] -> w247
            tunnel: [w357] -> w246
            tunnel: w241 -> [w347]
            tunnel: w234 -> [w348]
            tunnel: [w348] -> w233
            tunnel: [w347] -> w232
            tunnel: w266 -> [w406]
            tunnel: w263 -> [w419]
            tunnel: w260 -> [w412]
            tunnel: w259 -> [w411]
            tunnel: w258 -> [w410]
            tunnel: w257 -> [w409]
            tunnel: w255 -> [w418]
            tunnel: w253 -> [w417]
            tunnel: w236 -> [w415]
            tunnel: w243 -> [w416]
            tunnel: [w414] -> w249
            tunnel: [w413] -> w248
            tunnel: [w412] -> w237
            tunnel: [w411] -> w252
            tunnel: [w410] -> w251
            tunnel: [w409] -> w250
            tunnel: w247 -> [w408]
            tunnel: w246 -> [w407]
            tunnel: w233 -> [w404]
            tunnel: w232 -> [w403]
            frame #0 {
              n60 = Increment(x=w291) -> (x+1=w288:i32)
              n61 = case shown="True" w303 {
                tunnel: "Gap Refl1 (samples)" -> [_ w343]
                tunnel: w310 -> [w329 w339]
                tunnel: w308 -> [_ w336]
                tunnel: w306 -> [_ w342]
                tunnel: w294 -> [_ w341]
                tunnel: [w329 w340] -> w305
                tunnel: w297 -> [_ w338]
                tunnel: [dbl[] [] ("Locations") w337] -> w296
                tunnel: "Datenbank? R1-M1" -> [_ w335]
                tunnel: "Pfad? R1-M1" -> [_ w334]
                tunnel: w288 -> [_ w333]
                tunnel: "MaxtPeak miltiplication \nfactor -R1" -> [_ w332]
                tunnel: "Grenz Ampulitude-R1" -> [_ w331]
                tunnel: "Sigma-R1" -> [_ w330]
                frame False {
                }
                frame True {
                  n62 = call "Rangemap_Vi_BM_envelope_Huan_4.vi"("inputIR"=w336, "winkel"=w341, "distance from origin(cm) X"=w342, "Gap(samples)"=w343, "RangeMap"=w339, "MaxtPeak miltiplication factor"=w332, "distance from origin(cm) Y"=w338, "Datenbank?"=w335, "Grenz Ampulitude"=w331, "Pfad-Datenbank"=w334, "Wechle Lautsprecher?"=w333, "Sigma"=w330) -> ("Locations"=w337:dbl[], "OutputRangeMap2"=w340:dbl[][])  [unwired: 4 in, 2 out]
                }
              }
              n63 = case shown="True" w302 {
                tunnel: "Gap Refl1 (samples)" -> [_ w325]
                tunnel: w309 -> [w313 w324]
                tunnel: w307 -> [_ w327]
                tunnel: w306 -> [_ w323]
                tunnel: [w313 w320] -> w304
                tunnel: w294 -> [_ w322]
                tunnel: w297 -> [_ w321]
                tunnel: [dbl[] [] ("Locations") w326] -> w295
                tunnel: w288 -> [_ w319]
                tunnel: "Datenbank? R1-M2" -> [_ w318]
                tunnel: "Pfad? R1-M2" -> [_ w317]
                tunnel: "MaxtPeak miltiplication \nfactor -R1" -> [_ w316]
                tunnel: "Grenz Ampulitude-R1" -> [_ w315]
                tunnel: "Sigma-R1" -> [_ w314]
                frame False {
                }
                frame True {
                  n64 = call "Rangemap_Vi_BM_envelope_Huan_4.vi"("inputIR"=w327, "winkel"=w322, "distance from origin(cm) X"=w323, "Gap(samples)"=w325, "RangeMap"=w324, "MaxtPeak miltiplication factor"=w316, "distance from origin(cm) Y"=w321, "Datenbank?"=w318, "Grenz Ampulitude"=w315, "Pfad-Datenbank"=w317, "Wechle Lautsprecher?"=w319, "Sigma"=w314) -> ("Locations"=w326:dbl[], "OutputRangeMap2"=w320:dbl[][])  [unwired: 4 in, 2 out]
                }
              }
            }
            frame #1 {
              n65 = case shown="True" w357 {
                tunnel: "Gap Refl2 (samples)" -> [_ w381]
                tunnel: w365 -> [w368 w377]
                tunnel: w364 -> [_ w380]
                tunnel: w367 -> [_ w379]
                tunnel: [w368 w378] -> w360
                tunnel: w354 -> [_ w376]
                tunnel: w347 -> [_ w375]
                tunnel: w348 -> [_ w374]
                tunnel: "Datenbank? R2-M2" -> [_ w373]
                tunnel: "Pfad? R2-M2" -> [_ w372]
                tunnel: "MaxtPeak miltiplication\n factor -R2" -> [_ w371]
                tunnel: "Grenz Ampulitude-R2" -> [_ w370]
                tunnel: "Sigma-R2" -> [_ w369]
                frame False {
                }
                frame True {
                  n66 = call "Rangemap_Vi_BM_envelope_Huan_4.vi"("inputIR"=w380, "winkel"=w376, "distance from origin(cm) X"=w379, "Gap(samples)"=w381, "RangeMap"=w377, "MaxtPeak miltiplication factor"=w371, "distance from origin(cm) Y"=w375, "Datenbank?"=w373, "Grenz Ampulitude"=w370, "Pfad-Datenbank"=w372, "Wechle Lautsprecher?"=w374, "Sigma"=w369) -> ("OutputRangeMap2"=w378:dbl[][])  [unwired: 4 in, 3 out]
                }
              }
              n67 = case shown="True" w358 {
                tunnel: "Gap Refl2 (samples)" -> [_ w395]
                tunnel: w366 -> [w382 w391]
                tunnel: w353 -> [_ w394]
                tunnel: w367 -> [_ w390]
                tunnel: w354 -> [_ w393]
                tunnel: [w382 w392] -> w361
                tunnel: w347 -> [_ w389]
                tunnel: w348 -> [_ w388]
                tunnel: "Datenbank? R2-M1" -> [_ w387]
                tunnel: "Pfad? R2-M1" -> [_ w386]
                tunnel: "MaxtPeak miltiplication\n factor -R2" -> [_ w385]
                tunnel: "Grenz Ampulitude-R2" -> [_ w384]
                tunnel: "Sigma-R2" -> [_ w383]
                frame False {
                }
                frame True {
                  n68 = call "Rangemap_Vi_BM_envelope_Huan_4.vi"("inputIR"=w394, "winkel"=w393, "distance from origin(cm) X"=w390, "Gap(samples)"=w395, "RangeMap"=w391, "MaxtPeak miltiplication factor"=w385, "distance from origin(cm) Y"=w389, "Datenbank?"=w387, "Grenz Ampulitude"=w384, "Pfad-Datenbank"=w386, "Wechle Lautsprecher?"=w388, "Sigma"=w383) -> ("OutputRangeMap2"=w392:dbl[][])  [unwired: 4 in, 3 out]
                }
              }
            }
            frame #2 {
              n69 = case shown="True" w408 {
                tunnel: "Gap Refl3 (samples)" -> [_ w444]
                tunnel: w418 -> [w434 w443]
                tunnel: w416 -> [_ w447]
                tunnel: w419 -> [_ w445]
                tunnel: w406 -> [_ w446]
                tunnel: [w434 w442] -> w414
                tunnel: w404 -> [_ w441]
                tunnel: w403 -> [_ w440]
                tunnel: "Datenbank? R3-M1" -> [_ w439]
                tunnel: "Pfad? R3-M1" -> [_ w438]
                tunnel: "MaxtPeak miltiplication\n factor R3" -> [_ w437]
                tunnel: "Grenz Ampulitude-R3" -> [_ w436]
                tunnel: "Sigma-R3" -> [_ w435]
                frame False {
                }
                frame True {
                  n70 = call "Rangemap_Vi_BM_envelope_Huan_4.vi"("inputIR"=w447, "winkel"=w446, "distance from origin(cm) X"=w445, "Gap(samples)"=w444, "RangeMap"=w443, "MaxtPeak miltiplication factor"=w437, "distance from origin(cm) Y"=w440, "Datenbank?"=w439, "Grenz Ampulitude"=w436, "Pfad-Datenbank"=w438, "Wechle Lautsprecher?"=w441, "Sigma"=w435) -> ("OutputRangeMap2"=w442:dbl[][])  [unwired: 4 in, 3 out]
                }
              }
              n71 = case shown="True" w407 {
                tunnel: "Gap Refl3 (samples)" -> [_ w429]
                tunnel: w417 -> [w420 w430]
                tunnel: w415 -> [_ w432]
                tunnel: w419 -> [_ w428]
                tunnel: [w420 w433] -> w413
                tunnel: w406 -> [_ w431]
                tunnel: w404 -> [_ w427]
                tunnel: w403 -> [_ w426]
                tunnel: "Datenbank? R3-M2" -> [_ w425]
                tunnel: "Pfad? R3-M2" -> [_ w424]
                tunnel: "MaxtPeak miltiplication\n factor R3" -> [_ w423]
                tunnel: "Grenz Ampulitude-R3" -> [_ w422]
                tunnel: "Sigma-R3" -> [_ w421]
                frame False {
                }
                frame True {
                  n72 = call "Rangemap_Vi_BM_envelope_Huan_4.vi"("inputIR"=w432, "winkel"=w431, "distance from origin(cm) X"=w428, "Gap(samples)"=w429, "RangeMap"=w430, "MaxtPeak miltiplication factor"=w423, "distance from origin(cm) Y"=w426, "Datenbank?"=w425, "Grenz Ampulitude"=w422, "Pfad-Datenbank"=w424, "Wechle Lautsprecher?"=w427, "Sigma"=w421) -> ("OutputRangeMap2"=w433:dbl[][])  [unwired: 4 in, 3 out]
                }
              }
            }
          }
          n73 = stacked-sequence {
            seq-local: [w449 _ _] -> [_ w461 _]
            seq-local: [_ w464 _] -> [_ _ w470]
            seq-local: [_ _ w467] -> [_ _ _]
            seq-local: [w450 _ _] -> [_ w460 _]
            seq-local: [_ w462 _] -> [_ _ w469]
            seq-local: [_ _ w465] -> [_ _ _]
            tunnel: w284 -> [_ _ _]
            tunnel: w238 -> [w451 w463 _]
            tunnel: w235 -> [w448 _ _]
            tunnel: [_ _ w467] -> w283
            tunnel: [_ _ w465] -> w282
            tunnel: [_ _ w467] -> w243
            tunnel: [_ _ w465] -> w236
            frame #0 {
              # "Mic_2"
              # "Mic_1"
              n74 = call "synchronization_0.vi"("sweep signal"=w451) -> ("Micro 1/ ai 2"=w449:dbl[], "Micro 2/ai 1"=w450:dbl[])  [unwired: 9 in]
              n75 = case shown="True" "only one speaker" {
                tunnel: w448 -> [w457 _]
                tunnel: [w457 w458] -> w453
                frame False {
                }
                frame True {
                  n76 = Decrement(x="Numerisch") -> (x-1=w458:i32)
                }
              }
              n77 = call "sub_speaker_switch.vi"("Active Speaker\n(Index)"=w453, "Num of Speakers"=14, "task in"=refnum<k21> "Digital_14") -> ("Array (Ausgang)"=→"Active Speaker":bool[])  [unwired: 8 in]
            }
            frame #1 {
              # "Mic_2"
              # "Mic_1"
              # "Rohdaten Mic_2"
              # "Rohdaten Mic_1"
              n78 = call-poly <vilib>:"CrossCorrelation.vi"("Y"=w460, "X"=w463) -> ("Rxy"=w462:dbl[])  [unwired: 8 in, 1 out]
              "Mit Sweep korreliert 2" <- w462
              n79 = call-poly <vilib>:"CrossCorrelation.vi"("Y"=w461, "X"=w463) -> ("Rxy"=w464:dbl[])  [unwired: 8 in, 1 out]
              "Mit Sweep korreliert 1" <- w464
              "Rohdaten Mic_1" <- w461
              "Highpass gefilterte Rohdaten 1" <- w461
              "Rohdaten Mic_2" <- w460
              "Highpass gefilterte Rohdaten 2" <- w460
            }
            frame #2 {
              # "IR 1"
              # "IR 2"
              # "Gemittelte\nImpulsantworten 2"
              # "Mic_2"
              # "Korreliertes Signal 2"
              # "Mic_1"
              # "Gemittelte\nImpulsantworten 1"
              # "Korreliertes Signal 1"
              n80 = local read "Sequenz length us"() -> (w471:i32)
              n81 = Array Subset(array=w469, index="begin signal 2", length=w471) -> (w465:dbl[])
              "Korreliertes Signal mit richtigem Anfang 2" <- w465
              n82 = Array Subset(array=w470, index="begin signal 1", length=w471) -> (w467:dbl[])
              "Korreliertes Signal mit richtigem Anfang 1" <- w467
            }
          }
        }
        n83 = case shown="True" w218 {
          tunnel: w198 -> [_ w221]
          tunnel: w199 -> [_ w220]
          frame False {
          }
          frame True {
            w224 = "\\"
            w226 = "%s%s%s%s" ("format string")
            n84 = local read "Projektpfad"() -> (w225:path)
            n85 = local read "Projektname"() -> (w223:string)
            n86 = Format Into String(format string=w226, w225, w224, w223, "_ArrayRight.bin") -> (resulting string=w227:string)  [unwired: 2 in, 1 out]
            n87 = Format Into String(format string=w226, w225, w224, w223, "_ArrayLeft.bin") -> (resulting string=w230:string)  [unwired: 2 in, 1 out]
            n88 = String To Path(string=w227) -> (path=w228:path)
            n89 = String To Path(string=w230) -> (path=w229:path)
            n90 = Write to Binary File(file (use dialog)=w229, data=w221) -> ()  [unwired: 4 in, 3 out]
            n91 = Write to Binary File(file (use dialog)=w228, data=w220) -> ()  [unwired: 4 in, 3 out]
          }
        }
        n92 = call "singleChannelGraphs_1.vi"("Locations-IR 2"=w202, "Locations-IR 1"=w201, "micro 1"=w199, "micro 2"=w198) -> ()  [unwired: 8 in]
        n93 = call "Signal_SchrittfurSchritt.vi"("MaxtPeak miltiplication factor"="MaxtPeak miltiplication factor", "Standard Gap eingeben"="Standard Gap eingeben", "Mic.2"=w198, "Mic.1"=w199, "LS auswahlen"="LS auswählen", "Mic. auswählen"="Mic. 1      /      Mic. 2") -> ("Array 2"=→"Array 2":dbl[], "distanceMatrix"=→"distanceMatrix":dbl[][], "Locations"=→"Locations":dbl[], "IR with theshold"=→"Signalverlaufsgraph 3":dbl[][], "HS"=→"HS":bool, "korriliertes Signal"=→"korriliertes Singnal":dbl[])
      }
      frame #2 {
        # "Aktion Reflector 3 (blau)"
        # "Aktion Reflector 2 (blau)"
        # "Aktion Reflector 1 (orange)"
        n94 = Add(x=w560, y=w502) -> (x+y=w559:dbl[][])
        n95 = Add(x=w550, y=w549) -> (x+y=w552:dbl[][])
        n96 = Add(x=w503, y=w557) -> (x+y=w556:dbl[][])
        n97 = call "smooth 2D - x then y.vi"("2D array"=w559) -> ("x+y"=w558:dbl[][])  [unwired: 10 in]
        n98 = call "smooth 2D - x then y.vi"("2D array"=w552) -> ("x+y"=w551:dbl[][])  [unwired: 10 in]
        n99 = call "smooth 2D - x then y.vi"("2D array"=w556) -> ("x+y"=w555:dbl[][])  [unwired: 10 in]
        n100 = Add(x=w558, y=w501) -> (x+y=w478:dbl[][])
        "Refl_2" <- w478
        n101 = Add(x=w551, y=w546) -> (x+y=w525:dbl[][])
        "Refl_3" <- w525
        n102 = Add(x=w555, y=w554) -> (x+y=w528:dbl[][])
        "Refl_1" <- w528
        n103 = Array Max & Min(array=w525) -> (max value=w543:dbl, max index (indices)=w495:i32[])  [unwired: 2 out]
        n104 = Array Max & Min(array=w478) -> (max value=w544:dbl, max index (indices)=w494:i32[])  [unwired: 2 out]
        n105 = Array Max & Min(array=w528) -> (max value=w538:dbl, max index (indices)=w485:i32[])  [unwired: 2 out]
        n106 = Index Array(array=w495, index=1 ("Index")) -> (element=w547:i32)
        "y_R3" <- w547
        n107 = Subtract(x=w547, y=w486) -> (x-y=w483:dbl)
        "Abstand-Array-Refl3\n(in y Richtung)" <- w483
        n108 = Greater Than 0?(x=w483) -> (x > 0?=w496:bool)
        n109 = Index Array(array=w485, index=1 ("Index")) -> (element=w479:i32)
        "y_R1" <- w479
        n110 = Index Array(array=w494, index=1 ("Index")) -> (element=w480:i32)
        "y_R2" <- w480
        n111 = case shown="True" w496 {
          tunnel: w495 -> [_ w600]
          tunnel: w483 -> [w590 w595]
          tunnel: [w590 w591] -> w491
          frame False {
          }
          frame True {
            n112 = Square(x=w595) -> (x^2=w594:dbl)
            n113 = Index Array(array=w600, index=0 ("Index")) -> (element=w598:i32)
            "x_R3" <- w598
            n114 = Subtract(x=w598, y=100) -> (x-y=w596:i32)
            n115 = Square(x=w596) -> (x^2=w592:i32)
            n116 = Add(x=w594, y=w592) -> (x+y=w593:dbl)
            n117 = Square Root(x=w593) -> (sqrt(x)=w591:dbl)
          }
        }
        "Abstand-Array-Refl 3" <- w491
        n118 = Subtract(x=w479, y=w486) -> (x-y=w481:dbl)
        "Abstand-Array-Refl1\n(in y Richtung)" <- w481
        n119 = Subtract(x=w480, y=w486) -> (x-y=w482:dbl)
        "Abstand-Array-Refl2\n(in y Richtung)" <- w482
        n120 = Greater Than 0?(x=w482) -> (x > 0?=w493:bool)
        n121 = case shown="False" w493 {
          tunnel: w494 -> [w577 w589]
          tunnel: w482 -> [w579 w584]
          tunnel: [w579 w581] -> w492
          tunnel: [w576 w580] -> w490
          frame False {
            n122 = Index Array(array=w577, index=0 ("Index")) -> (element=w576:i32)
            "x_R2" <- w576
          }
          frame True {
            n123 = Index Array(array=w589, index=0 ("Index")) -> (element=w580:i32)
            n124 = Square(x=w584) -> (x^2=w583:dbl)
            n125 = Subtract(x=w580, y=100) -> (x-y=w586:i32)
            n126 = Square(x=w586) -> (x^2=w585:i32)
            n127 = Add(x=w583, y=w585) -> (x+y=w582:dbl)
            n128 = Square Root(x=w582) -> (sqrt(x)=w581:dbl)
          }
        }
        "Abstand-Array-Refl 2" <- w492
        n129 = Greater Than 0?(x=w481) -> (x > 0?=w484:bool)
        n130 = case shown="True" w484 {
          tunnel: [w565 w570] -> w487
          tunnel: w481 -> [w565 w569]
          tunnel: w485 -> [_ w567]
          frame False {
          }
          frame True {
            n131 = Index Array(array=w567, index=0 ("Index")) -> (element=w566:i32)
            "x_R1" <- w566
            n132 = Subtract(x=w566, y=100) -> (x-y=w575:i32)
            n133 = Square(x=w575) -> (x^2=w568:i32)
            n134 = Square(x=w569) -> (x^2=w571:dbl)
            n135 = Add(x=w571, y=w568) -> (x+y=w572:dbl)
            n136 = Square Root(x=w572) -> (sqrt(x)=w570:dbl)
          }
        }
        "Abstand-Array-Refl1" <- w487
        n137 = local read "Actions?"() -> (w513:bool)
        n138 = Less Or Equal?(x=w490, y=100) -> (x <= y?=w489:bool)
        n139 = Build Array (concatenate)(w545, w543) -> (w473:dbl[])
        n140 = Array Size(array=w473) -> (size(s)=w533:i32)
        n141 = Subtract(x=w533, y=2) -> (x-y=w531:i32)
        n142 = Array Subset(array=w473, index=w531) -> (w530:dbl[])  [unwired: 1 in]
        n143 = Build Array (concatenate)(w561, w544) -> (w474:dbl[])
        n144 = Array Size(array=w474) -> (size(s)=w537:i32)
        n145 = Subtract(x=w537, y=2) -> (x-y=w535:i32)
        n146 = Array Subset(array=w474, index=w535) -> (w534:dbl[])  [unwired: 1 in]
        n147 = Build Array (concatenate)(w562, w538) -> (w529:dbl[])
        n148 = Array Size(array=w529) -> (size(s)=w542:i32)
        n149 = Subtract(x=w542, y=2) -> (x-y=w540:i32)
        n150 = Array Subset(array=w529, index=w540) -> (w539:dbl[])  [unwired: 1 in]
        n151 = call-poly <vilib>:"Mean.vi"("X"=w539) -> ("mean"=w522:dbl)  [unwired: 1 out]
        "Max. Wert Refl_1" <- w522
        n152 = call-poly <vilib>:"Mean.vi"("X"=w534) -> ("mean"=w520:dbl)  [unwired: 1 out]
        "Max. Wert Refl_2" <- w520
        n153 = call-poly <vilib>:"Mean.vi"("X"=w530) -> ("mean"=w497:dbl)  [unwired: 1 out]
        "Max. Wert Refl_3" <- w497
        n154 = call "Decider_BM_schwelle_dist_Huan.vi"("Max. Wert Refl_1"=w522, "Abstand-Array-Refl 1"=w481, "stop abstand 1"="Stopabstand 1", "Max. Wert Refl_2"=w520, "Abstand-Array-Refl 2"=w482, "stop abstand 2"="Stopabstand 2", "Max. Wert Refl_3"=w497, "Abstand-Array-Refl 3"=w483, "stop abstand 3"="Stopabstand 3") -> ("R1-action"=w517:bool, "R2-action"=w516:bool, "R3-action"=w500:bool, "Prop 1"=w511:dbl, "Prop 2"=w510:dbl, "Prop 3"=w509:dbl)  [unwired: 5 in]
        "R1-Action" <- w517
        "R2-Action" <- w516
        "R3-Action" <- w500
        n155 = Compound Arithmetic op=AND(w513, w516, "turn left/right?") -> (w505:bool)
        n156 = Compound Arithmetic op=AND(w513, w500, "LED turn on?") -> (w499:bool)
        n157 = case shown="True" w499 {
          tunnel: w525 -> [w601 _]
          tunnel: [w601 w602] -> w524
          tunnel: w472 -> [_ w603]
          frame False {
          }
          frame True {
            n158 = flat-sequence {
              tunnel: w603 -> [w613]
              tunnel: [w613] -> w602
              frame #0 {
                n159 = call-poly <vilib>:"DAQmx Write.vi"("task/channels in"=refnum<k21> "LED", "data"=TRUE) -> ("task out"=w612:refnum<k21>, "error out"=w611:errorcluster)  [unwired: 11 in, 1 out]
                n160 = call <vilib>:"DAQmx Start Task.vi"("task/channels in"=w612, "error in"=w611) -> ("task out"=w610:refnum<k21>, "error out"=w609:errorcluster)  [unwired: 12 in]
                n161 = call <vilib>:"DAQmx Is Task Done.vi"("task/channels in"=w610, "error in"=w609) -> ("task out"=w608:refnum<k21>, "error out"=w607:errorcluster)  [unwired: 11 in, 1 out]
                n162 = call <vilib>:"DAQmx Stop Task.vi"("task/channels in"=w608, "error in"=w607) -> ("error out"=→"error out 7":errorcluster)  [unwired: 12 in, 1 out]
              }
              frame #1 {
                n163 = local write "LED turn on?"(FALSE) -> ()
              }
            }
          }
        }
        n164 = case shown="True" w505 {
          tunnel: w478 -> [w616 _]
          tunnel: [w616 w618] -> w526
          tunnel: w489 -> [_ w620]
          tunnel: w472 -> [_ w619]
          frame False {
            n165 = local write "turn left/right?"(TRUE) -> ()
          }
          frame True {
            n166 = flat-sequence {
              tunnel: w620 -> [w622]
              tunnel: w619 -> [w621]
              tunnel: [w621] -> w617
              tunnel: [w682] -> w618
              tunnel: w617 -> [w682]
              frame #0 {
                n167 = case shown="False" w622 {
                  frame False {
                    n168 = flat-sequence {
                      tunnel: [w629] -> w627
                      tunnel: w627 -> [w632]
                      tunnel: [w632] -> w626
                      tunnel: w626 -> [w643]
                      tunnel: [w643] -> w625
                      tunnel: [w635] -> w624
                      tunnel: w625 -> [w648]
                      tunnel: [w648] -> w623
                      tunnel: w624 -> [w647]
                      tunnel: w623 -> [w651]
                      frame #0 {
                        w629 = refnum<visa-resource-name> "COM4" ("VISA resource name")
                        # "left turn"
                        n169 = call "sub_EasyIsel.vi"("VISA resource name"=w629, "Mode"=enum16{"Position", "Move", "Stop", "Home"}."Stop") -> ()  [unwired: 14 in, 4 out]
                        n170 = Wait (ms)(milliseconds to wait=u32 100 ("Zu wartende ms")) -> ()  [unwired: 1 out]
                      }
                      frame #1 {
                        n171 = Wait (ms)(milliseconds to wait=u32 1000 ("Zu wartende ms")) -> ()  [unwired: 1 out]
                      }
                      frame #2 {
                        w639 = 157.0 ("Steps/mm (z)")
                        w640 = 3000.0 ("Velocity (z)")
                        w638 = -100.0 ("z-Position")
                        n172 = Divide(x=w640, y=w639) -> (x/y=w636:dbl)
                        n173 = Absolute Value(x=w638) -> (abs(x)=w637:dbl)
                        n174 = local read "origin Y(cm)"() -> (w633:dbl)
                        n175 = call "sub_EasyIsel.vi"("z-Position"=w638, "Velocity (z)"=w640, "VISA resource name"=w643, "Mode"=enum16{"Position", "Move", "Stop", "Home"}."Move", "Steps/mm (z)"=w639) -> ()  [unwired: 11 in, 4 out]
                        n176 = Divide(x=w637, y=w636) -> (x/y=w635:dbl)
                        n177 = Divide(x=w638, y=10.0 ("x/y")) -> (x/y=w641:dbl)
                        n178 = Add(x=w641, y=w633) -> (x+y=w634:dbl)
                        n179 = local write "origin Y(cm)"(w634) -> ()
                      }
                      frame #3 {
                        n180 = Multiply(x=u32 1000 ("Zu wartende ms"), y=w647) -> (x*y=w645:dbl)
                        n181 = Wait (ms)(milliseconds to wait=w645) -> ()  [unwired: 1 out]
                      }
                      frame #4 {
                        n182 = local read "x-move (mm)"() -> (w649:dbl)
                        n183 = local read "Velocity"() -> (w650:dbl)
                        n184 = call "sub_EasyIsel.vi"("x-Position"=w649, "Velocity (x)"=w650, "VISA resource name"=w651, "Mode"=enum16{"Position", "Move", "Stop", "Home"}."Move") -> ()  [unwired: 12 in, 4 out]
                      }
                    }
                  }
                  frame True {
                    n185 = flat-sequence {
                      tunnel: [w659] -> w657
                      tunnel: w657 -> [w662]
                      tunnel: [w662] -> w656
                      tunnel: w656 -> [w672]
                      tunnel: [w672] -> w655
                      tunnel: [w665] -> w654
                      tunnel: w655 -> [w677]
                      tunnel: [w677] -> w653
                      tunnel: w654 -> [w675]
                      tunnel: w653 -> [w680]
                      frame #0 {
                        w659 = refnum<visa-resource-name> "COM4" ("VISA resource name")
                        # "right turn"
                        n186 = call "sub_EasyIsel.vi"("VISA resource name"=w659, "Mode"=enum16{"Position", "Move", "Stop", "Home"}."Stop") -> ()  [unwired: 14 in, 4 out]
                        n187 = Wait (ms)(milliseconds to wait=u32 100 ("Zu wartende ms")) -> ()  [unwired: 1 out]
                      }
                      frame #1 {
                        n188 = Wait (ms)(milliseconds to wait=u32 1000 ("Zu wartende ms")) -> ()  [unwired: 1 out]
                      }
                      frame #2 {
                        w668 = 157.0 ("Steps/mm (z)")
                        w669 = 3000.0 ("Velocity (z)")
                        w667 = 100.0 ("z-Position")
                        n189 = local read "origin Y(cm)"() -> (w664:dbl)
                        n190 = Divide(x=w669, y=w668) -> (x/y=w666:dbl)
                        n191 = call "sub_EasyIsel.vi"("z-Position"=w667, "Velocity (z)"=w669, "VISA resource name"=w672, "Mode"=enum16{"Position", "Move", "Stop", "Home"}."Move", "Steps/mm (z)"=w668) -> ()  [unwired: 11 in, 4 out]
                        n192 = Divide(x=w667, y=10.0 ("x/y")) -> (x/y=w670:dbl)
                        n193 = Divide(x=w667, y=w666) -> (x/y=w665:dbl)
                        n194 = Add(x=w670, y=w664) -> (x+y=w663:dbl)
                        n195 = local write "origin Y(cm)"(w663) -> ()
                      }
                      frame #3 {
                        n196 = Multiply(x=1000.0, y=w675) -> (x*y=w674:dbl)
                        n197 = Wait (ms)(milliseconds to wait=w674) -> ()  [unwired: 1 out]
                      }
                      frame #4 {
                        n198 = local read "x-move (mm)"() -> (w678:dbl)
                        n199 = local read "Velocity"() -> (w679:dbl)
                        n200 = call "sub_EasyIsel.vi"("x-Position"=w678, "Velocity (x)"=w679, "VISA resource name"=w680, "Mode"=enum16{"Position", "Move", "Stop", "Home"}."Move") -> ()  [unwired: 12 in, 4 out]
                      }
                    }
                  }
                }
              }
              frame #1 {
                n201 = local write "turn left/right?"(FALSE) -> ()
              }
            }
            n202 = flat-sequence {
              frame #0 {
                n203 = local write "Message"("0;7;15" ("Message")) -> ()
                n204 = Wait (ms)(milliseconds to wait=u32 3000 ("Zu wartende ms")) -> ()  [unwired: 1 out]
              }
              frame #1 {
                n205 = local write "Message"("60;0;15" ("Message")) -> ()
              }
            }
          }
        }
        n206 = Build Array (concatenate)(w506, w509) -> (w475:dbl[])
        n207 = Build Array (concatenate)(w507, w511) -> (w508:dbl[])
        n208 = Build Array (concatenate)(w477, w510) -> (w476:dbl[])
        n209 = Compound Arithmetic op=AND(w513, w517) -> (w504:bool)
        n210 = Build Array(w508, w475, w476) -> (→"probability/distance":dbl[][])
        n211 = Build Array(w529, w473, w474) -> (→"probability":dbl[][])
        n212 = case shown="True" w504 {
          tunnel: [FALSE TRUE] -> w498
          tunnel: w528 -> [w687 _]
          tunnel: [w687 w701] -> w527
          tunnel: w472 -> [_ w701]
          frame False {
          }
          frame True {
            n213 = call-poly <vilib>:"DAQmx Write.vi"("task/channels in"=refnum<k21> "LED", "data"=FALSE) -> ("task out"=w700:refnum<k21>, "error out"=w699:errorcluster)  [unwired: 11 in, 1 out]
            n214 = Initialize Array(FALSE, 14 ("dimension size")) -> (w712:bool[])
            n215 = call "sub_EasyIsel.vi"("VISA resource name"=refnum<visa-resource-name> "COM4", "Mode"=enum16{"Position", "Move", "Stop", "Home"}."Stop") -> ()  [unwired: 14 in, 4 out]
            n216 = call <vilib>:"DAQmx Start Task.vi"("task/channels in"=w700, "error in"=w699) -> ("task out"=w698:refnum<k21>, "error out"=w697:errorcluster)  [unwired: 12 in]
            n217 = call-poly <vilib>:"DAQmx Write.vi"("task/channels in"=refnum<k21> "Digital_14" ("task in"), "data"=w712) -> ("task out"=w702:refnum<k21>, "error out"=w703:errorcluster)  [unwired: 11 in, 1 out]
            n218 = call <vilib>:"DAQmx Is Task Done.vi"("task/channels in"=w698, "error in"=w697) -> ("task out"=w696:refnum<k21>, "error out"=w695:errorcluster)  [unwired: 11 in, 1 out]
            n219 = call <vilib>:"DAQmx Start Task.vi"("task/channels in"=w702, "error in"=w703) -> ("task out"=w704:refnum<k21>, "error out"=w705:errorcluster)  [unwired: 12 in]
            n220 = call <vilib>:"DAQmx Stop Task.vi"("task/channels in"=w696, "error in"=w695) -> ("error out"=→"error out 6":errorcluster)  [unwired: 12 in, 1 out]
            n221 = call <vilib>:"DAQmx Is Task Done.vi"("task/channels in"=w704, "error in"=w705) -> ("task out"=w706:refnum<k21>, "error out"=w707:errorcluster)  [unwired: 11 in, 1 out]
            n222 = call <vilib>:"DAQmx Stop Task.vi"("task/channels in"=w706, "error in"=w707) -> ("error out"=→"error out 2":errorcluster)  [unwired: 12 in, 1 out]
            n223 = local write "Message"("0;0;15" ("Message")) -> ()
          }
        }
      }
    }
    n224 = case shown="True" w84 {
      tunnel: w98 -> [w149 _]
      tunnel: [w149 w150] -> w97
      frame False {
      }
      frame True {
        n225 = Get Date/Time In Seconds() -> (seconds since 1Jan1904=w150:timestamp)
      }
    }
    n226 = local read "Stopp 2"() -> (w80:bool)
    n227 = Or(x=w79, y=w80) -> (x .or. y?=w78:bool)
    n228 = case shown="True" w78 {
      frame False {
      }
      frame True {
        n229 = call "sub_EasyIsel.vi"("VISA resource name"=refnum<visa-resource-name> "COM4", "Mode"=enum16{"Position", "Move", "Stop", "Home"}."Stop") -> ()  [unwired: 14 in, 4 out]
      }
    }
  }
